vi "Resolve VI Path.vi"(8 "error in (no error)":errorcluster, 10 "Library Paths (.lvlibp, .lvlib)":path[](array[path]), 11 "Qualified Name (lvlibp|lvlib[:vi])":string) -> (0 "error out":errorcluster, 3 "VI Path":path)   [LabVIEW 2022 SP3, in "Core.lvlib" / "Config.lvlib"]
uses:
  Config.lvlib
  <vilib>/Utility/LVLibp/NI_PackedLibraryUtility.lvlib
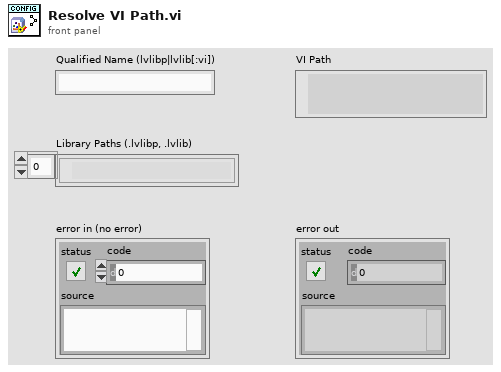
[diagram p1: front panel]
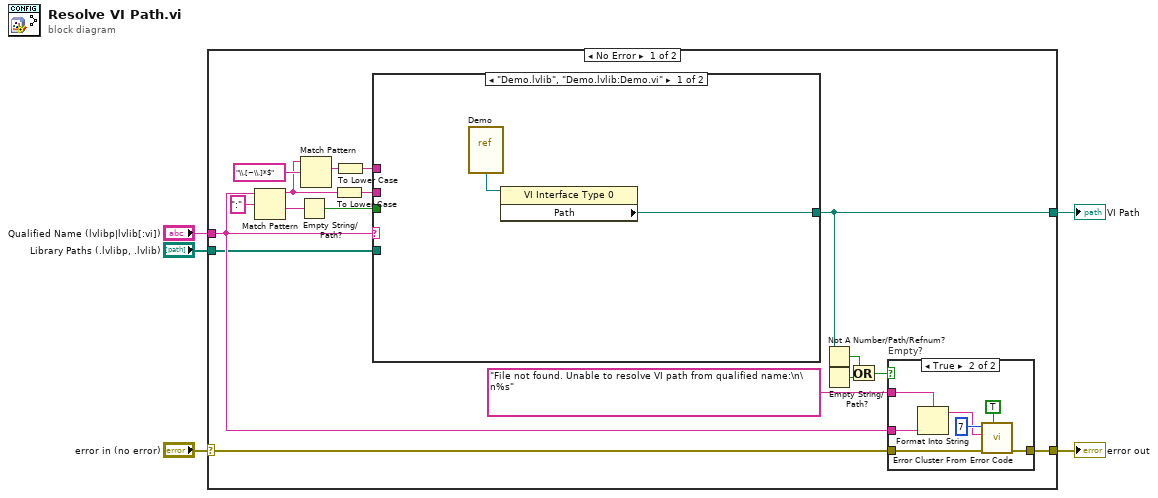
[diagram p0: block diagram]
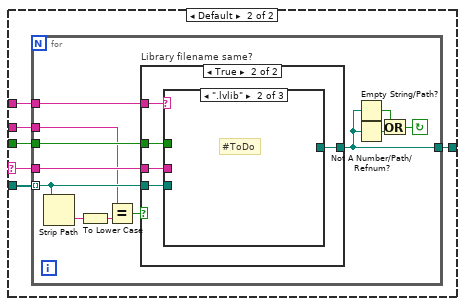
[diagram p2: hidden frame]
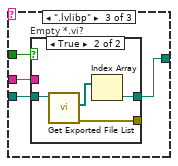
[diagram p5: hidden frame]
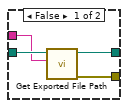
[diagram p6: hidden frame]
diagram:
  n1 = case shown="No Error" "error in (no error)" {
    selector: "error in (no error)" -> [w15 w68]
    tunnel: "Qualified Name (lvlibp|lvlib[:vi])" -> [w10 _]
    tunnel: [w14 w68] -> w3
    tunnel: "Library Paths (.lvlibp, .lvlib)" -> [w7 _]
    tunnel: [w11 _] -> w1
    frame No Error {
      n2 = Match Pattern(string=w10, regular expression=":") -> (before substring=w20:string, after substring=w17:string)  [unwired: 1 in, 2 out]
      n3 = Empty String/Path?(string/path=w17) -> (empty?=w16:bool)
      n4 = Match Pattern(string=w20, regular expression="\\.[~\\.]*$") -> (match substring=w19:string)  [unwired: 4 out]
      n5 = To Lower Case(string=w20) -> (all lower case string=w6:string)
      n6 = To Lower Case(string=w19) -> (all lower case string=w18:string)
      n7 = case shown="\"Demo.lvlib\", \"Demo.lvlib:Demo.vi\"" w10 {
        selector: w10 -> [_ w26]
        tunnel: w6 -> [_ w25]
        tunnel: w7 -> [_ w30]
        tunnel: w18 -> [_ w29]
        tunnel: w16 -> [_ w28]
        tunnel: [w24 w27] -> w11
        frame "Demo.lvlib", "Demo.lvlib:Demo.vi" {
          n8 = vi-ref "Demo.vi"() -> (w23:refnum<vi>)
          n9 = property class="VI Interface Type 0"(reference=w23) -> ("Path"=w24:path)  [unwired: 1 in, 2 out]
        }
        frame Default {
          n10 = for {
            tunnel: w26 -> [w42]
            tunnel: w28 -> [w41]
            tunnel: [w33] -> w27
            tunnel: w29 -> [w37]
            tunnel: w30 -> [w40] mode=indexing
            tunnel: w25 -> [w31]
            stop <- w32 continue-if-true
            n11 = Strip Path(path=w40) -> (name=w39:string)  [unwired: 1 out]
            n12 = To Lower Case(string=w39) -> (all lower case string=w38:string)
            n13 = Equal?(x=w31, y=w38) -> (x = y?=w36:bool)
            n14 = case "Library filename same?" shown="True" w36 {
              tunnel: w42 -> [_ w46]
              tunnel: w41 -> [_ w44]
              tunnel: [_ w45] -> w33
              tunnel: w40 -> [_ w47]
              tunnel: w37 -> [_ w43]
              frame False {
              }
              frame True {
                n15 = case shown="\".lvlib\"" w43 {
                  tunnel: w47 -> [_ _ w51]
                  tunnel: w46 -> [_ _ w50]
                  tunnel: [_ _ w49] -> w45
                  tunnel: w44 -> [_ _ w48]
                  frame Default {
                  }
                  frame ".lvlib" {
                    # "#ToDo"
                  }
                  frame ".lvlibp" {
                    n16 = case "Empty *.vi?" shown="True" w48 {
                      tunnel: w51 -> [w55 w59]
                      tunnel: w50 -> [w54 _]
                      tunnel: [w53 w57] -> w49
                      tunnel: [w52 w56] -> _
                      frame False {
                        n17 = call <vilib>:"Get Exported File Path.vi"("qualified name"=w54, "packed library path"=w55) -> ("error out"=w52:errorcluster, "path"=w53:path)  [unwired: 8 in]
                      }
                      frame True {
                        n18 = call <vilib>:"Get Exported File List.vi"("packed library path"=w59) -> ("error out"=w56:errorcluster, "paths"=w58:path[])  [unwired: 8 in, 1 out]
                        n19 = Index Array(array=w58) -> (element=w57:path)  [unwired: 1 in]
                      }
                    }
                  }
                }
              }
            }
            n20 = Empty String/Path?(string/path=w33) -> (empty?=w34:bool)
            n21 = Not A Number/Path/Refnum?(number/path/refnum=w33) -> (NaN/Path/Refnum?=w35:bool)
            n22 = Or(x=w34, y=w35) -> (x .or. y?=w32:bool)
          }
        }
      }
      n23 = Not A Number/Path/Refnum?(number/path/refnum=w11) -> (NaN/Path/Refnum?=w13:bool)
      n24 = Empty String/Path?(string/path=w11) -> (empty?=w12:bool)
      n25 = Or(x=w13, y=w12) -> (x .or. y?=w8:bool)
      n26 = case "Empty?" shown="True" w8 {
        tunnel: w15 -> [w60 w67]
        tunnel: [w60 w66] -> w14
        tunnel: w10 -> [_ w63]
        tunnel: "File not found. Unable to resolve VI path from qualified name:\n\n%s" ("format string") -> [_ w62]
        frame False {
        }
        frame True {
          n27 = Format Into String(format string=w62, w63) -> (resulting string=w61:string)  [unwired: 2 in, 1 out]
          n28 = call <vilib>:"Error Cluster From Error Code.vi"("show call chain? (False)"=TRUE, "error in (no error)"=w67, "error message (\"\")"=w61, "error code (0)"=7) -> ("error out"=w66:errorcluster)  [unwired: 5 in]
        }
      }
    }
    frame Error {
    }
  }
  "error out" <- w3
  "VI Path" <- w1
